vi "QQQQQQ.vi"(1 "Q":dbl) -> (0 "proni":dbl)   [LabVIEW 2018]
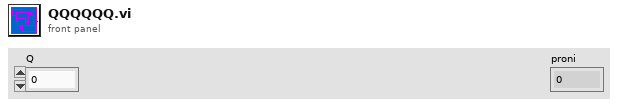
[diagram p1: front panel]
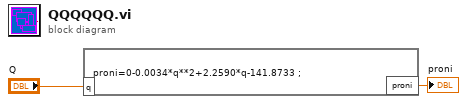
[diagram p0: block diagram]
diagram:
  n1 = formula code="proni=0-0.0034*q**2+2.2590*q-141.8733 ;"("q"="Q") -> ("proni"=→"proni":dbl)
